vi "Signal_with_time_information.vi"() -> ()   [LabVIEW 2017]
panel:
  out "Signal with time":waveform(i32)(graph)
  in  "stop":bool
  in  "Samples qty":i32
  in  "Period (ms)":u32=10
  in  "COM Port":refnum<visa-resource-name>="COM1"
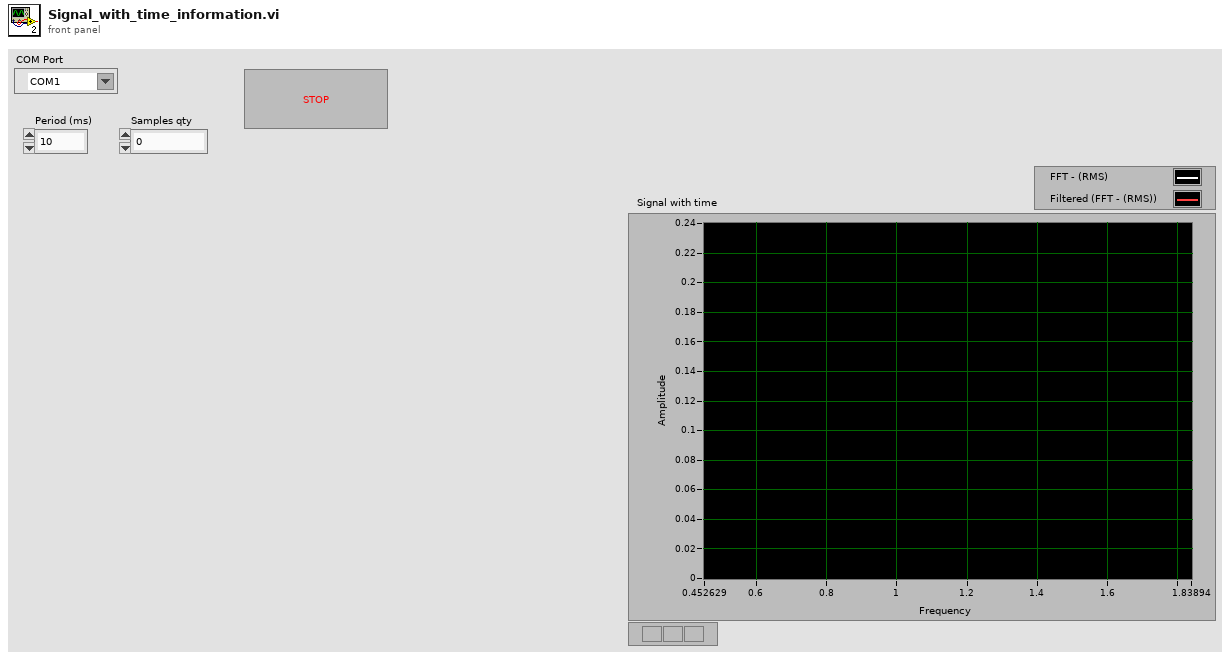
[diagram p1: front panel]
types:
  T1 = typedef "device.ctl" = cluster{"Device Session":refnum<visa-resource-name>, "dT":i32}
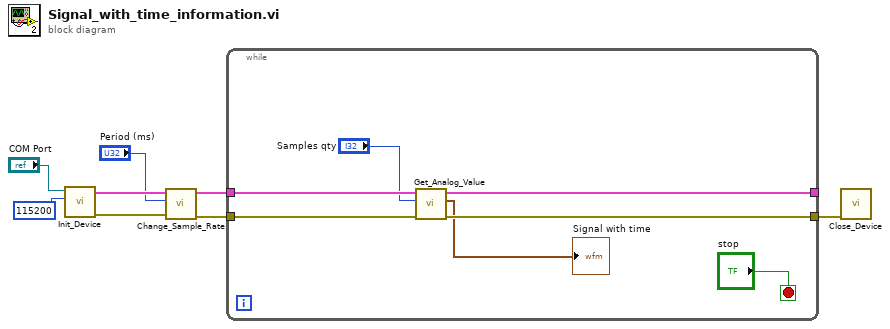
[diagram p0: block diagram]
diagram:
  n1 = call "Init_Device.vi"("Baud Rate (115200)"=u32 115200 ("Baud Rate"), "COM Port"="COM Port") -> ("error out"=w5:errorcluster, "Device"=w6:T1)  [unwired: 8 in]
  n2 = call "Change_Sample_Rate.vi"("error in"=w5, "Period [ms]"="Period (ms)", "Device IN"=w6) -> ("error out"=w4:errorcluster, "Device OUT"=w3:T1)  [unwired: 7 in]
  n3 = while {
    tunnel: w4 -> [w15]
    tunnel: w3 -> [w14]
    tunnel: [w11] -> w2
    tunnel: [w10] -> _
    stop <- "stop" stop-if-true
    n4 = call "Get_Analog_Value.vi"("error in"=w15, "Samples qty (1)"="Samples qty", "Device IN"=w14) -> ("error out"=w11:errorcluster, "output waveform"=→"Signal with time":waveform(i32), "Device OUT"=w10:T1)  [unwired: 5 in]
  }
  n5 = call "Close_Device.vi"("error in"=w2) -> ()  [unwired: 9 in, 1 out]
